vi "Finish.vi"   [LabVIEW 2012]
doc: "This VI is called just before exiting. It is expected to close I/O refnum, save collected data, etc."
uses:
  <vilib>/Rock Robotics/WPI/Compressor/WPI_CompressorGetSetRefNum.vi
  <vilib>/Rock Robotics/WPI/Joystick/WPI_JoystickGetSetRefNum.vi
  <vilib>/Rock Robotics/WPI/RobotDrive/WPI_RobotDriveGetSetRefNum.vi
types:
  T1 = typedef "WPI_ServoDeviceRef.ctl" = cluster{"DeviceStatus":errorcluster, "Digital Module":T2, "PWM Channel":T3, "DeadBand":T4}
  T2 = typedef "FPGA_TypedefDigitalModule.ctl" = enum16{"Digital Module 1", "Digital Module 2"}
  T3 = typedef "FPGA_DIOPWMChannel.ctl" = enum8{"PWM 1", "PWM 2", "PWM 3", "PWM 4", "PWM 5", "PWM 6", "PWM 7", "PWM 8", "PWM 9", "PWM 10", "Invalid"}
  T4 = typedef "WPI_PWMDeadband.ctl" = cluster{"Name":string, "maxPositivePwm":i32, "minPositivePwm":i32, "centerPwm":i32, "maxNegativePwm":i32, "minNegativePwm":i32, "angularRange":u16}
  T5 = typedef "WPI_JoystickDevRef.ctl" = cluster{"Device":T6}
  T6 = typedef "WPI_JoystickDeviceEnum.ctl" = enum16{"USB 1", "USB 2", "USB 3", "USB 4", "Kinect 1", "Kinect 2"}
  T7 = typedef "WPI_RobotDriveDevRef.ctl" = cluster{"DevStatus":errorcluster, "Motors[]":T8[], "Square Inputs":bool, "Max Output":dbl, "Isochronous":bool}
  T8 = typedef "WPI_MotorControlDeviceRef.ctl" = cluster{"DeviceStatus":errorcluster, "Type":enum16{"PWM", "CAN"}, "PWM":cluster{"Digital Module":T2, "PWM Channel":T3, "DeadBand":T4}, "CAN":cluster{"Device Number":u8, "Control Mode":T9, "Semaphore":T10, "Max Vout":dbl}, "Invert":bool, "TransformRef":T11, "InvTransformRef":T11}
  T9 = typedef "WPI_CANJaguar_ControlMode.ctl" = enum8{"Percent VBus", "Current", "Speed", "Position", "Voltage"}
  T10 = typedef "Semaphore RefNum" = refnum<k1>
  T11 = typedef "WPI_PWMTransform_ConPane.ctl" = refnum<vi>
  T12 = typedef "WPI_SolenoidDevRef.ctl" = cluster{"DevStatus":errorcluster, "Solenoid Module":T13, "Forward Solenoid Channel":T14, "Reverse Solenoid Channel":T14}
  T13 = typedef "FPGA_TypedefSolenoidModule.ctl" = enum16{"Solenoid Module 1", "Solenoid Module 2"}
  T14 = typedef "WPI_SolenoidChannel.ctl" = enum8{"Solenoid 1", "Solenoid 2", "Solenoid 3", "Solenoid 4", "Solenoid 5", "Solenoid 6", "Solenoid 7", "Solenoid 8", "Invalid"}
  T15 = typedef "WPI_EncoderDevRef.ctl" = cluster{"DevStatus":errorcluster, "EncoderIndex":T16, "CounterIndex":T17, "DistancePerCount":dbl, "Decoding Type":T18}
  T16 = typedef "FPGA_EncoderIdx.ctl" = enum8{"Enc 0", "Enc 1", "Enc 2", "Enc 3", "Invalid"}
  T17 = typedef "FPGA_CounterCtrSystemIndex.ctl" = enum8{"Ctr 0", "Ctr 1", "Ctr 2", "Ctr 3", "Ctr 4", "Ctr 5", "Ctr 6", "Ctr 7", "Invalid"}
  T18 = typedef "WPI_EncoderType.ctl" = enum16{"1x", "2x", "4x"}
  T19 = typedef "WPI_GyroDevRef.ctl" = cluster{"DevStatus":errorcluster, "Analog Module":T20, "Analog Channel":T21, "Offset":dbl, "Gain (VoltsPerDegree/Second)":dbl}
  T20 = typedef "FPGA_TypedefAnalogModule.ctl" = enum16{"Analog Module 1", "Analog Module 2"}
  T21 = typedef "FPGA_AIChannel.ctl" = enum8{"AI 1", "AI 2", "AI 3", "AI 4", "AI 5", "AI 6", "AI 7", "AI 8", "Invalid"}
  T22 = typedef "WPI_DigitalInputDevRef.ctl" = cluster{"DevStatus":errorcluster, "DIO Channel":T23, "Digital Module":T2}
  T23 = typedef "FPGA_DIOChannel.ctl" = enum8{"DIO 1", "DIO 2", "DIO 3", "DIO 4", "DIO 5", "DIO 6", "DIO 7", "DIO 8", "DIO 9", "DIO 10", "DIO 11", "DIO 12", "DIO 13", "DIO 14", "Invalid"}
  T24 = typedef "WPI_CompressorDevRef.ctl" = cluster{"DevStatus":errorcluster, "DigitalInputDevRef":T22, "RelayDevRef":T25}
  T25 = typedef "WPI_RelayDevRef.ctl" = cluster{"DevStatus":errorcluster, "Relay Channel":T26, "Digital Module":T2, "Relay Direction":T27}
  T26 = typedef "FPGA_DIORelayChannel.ctl" = enum8{"Relay 1", "Relay 2", "Relay 3", "Relay 4", "Relay 5", "Relay 6", "Relay 7", "Relay 8", "Invalid"}
  T27 = typedef "WPI_RelayDirection.ctl" = enum16{"Both directions", "Forward only", "Reverse only"}
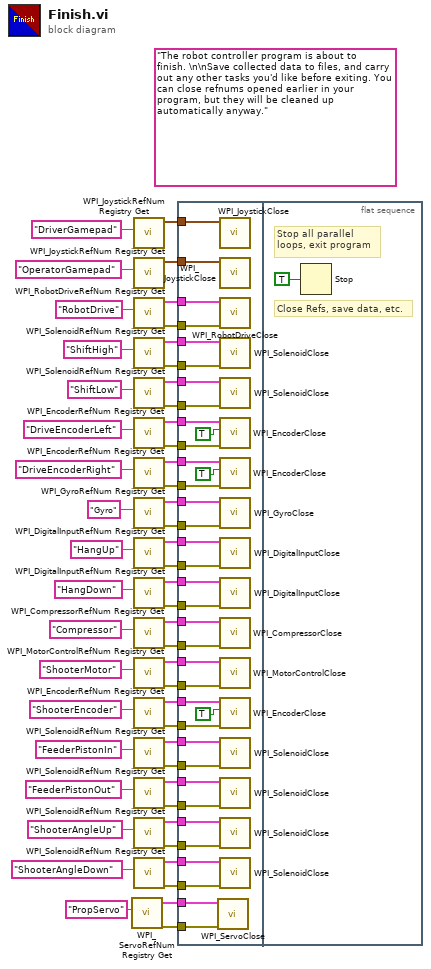
[diagram p0: block diagram]
diagram:
  (unwired) "The robot controller program is about to finish. \n\nSave collected data to files, and carry out any other tasks you'd like before exiting. You can close refnums opened earlier in your program, but they will be cleaned up automatically anyway."
  n1 = call <vilib>:"WPI_ServoRefNum Registry Get.vi"("refnum name"="PropServo") -> ("error out"=w1:errorcluster, "ServoDeviceRef"=w2:T1)  [unwired: 9 in]
  n2 = call <vilib>:"WPI_JoystickRefNum Registry Get.vi"("refnum name"="DriverGamepad") -> ("JoystickDevRef"=w35:T5)  [unwired: 1 in, 9 out]
  n3 = call <vilib>:"WPI_JoystickRefNum Registry Get.vi"("refnum name"="OperatorGamepad") -> ("JoystickDevRef"=w34:T5)  [unwired: 1 in, 9 out]
  n4 = call <vilib>:"WPI_RobotDriveRefNum Registry Get.vi"("refnum name"="RobotDrive") -> ("error out"=w31:errorcluster, "RobotDriveDevRef"=w33:T7)  [unwired: 1 in, 8 out]
  n5 = call <vilib>:"WPI_SolenoidRefNum Registry Get.vi"("refnum name"="ShiftHigh") -> ("error out"=w30:errorcluster, "SolenoidDevRef"=w32:T12)  [unwired: 9 in]
  n6 = call <vilib>:"WPI_SolenoidRefNum Registry Get.vi"("refnum name"="ShiftLow") -> ("error out"=w28:errorcluster, "SolenoidDevRef"=w29:T12)  [unwired: 9 in]
  n7 = call <vilib>:"WPI_EncoderRefNum Registry Get.vi"("refnum name"="DriveEncoderLeft") -> ("error out"=w26:errorcluster, "EncoderDevRef"=w27:T15)  [unwired: 9 in]
  n8 = call <vilib>:"WPI_EncoderRefNum Registry Get.vi"("refnum name"="DriveEncoderRight") -> ("error out"=w22:errorcluster, "EncoderDevRef"=w23:T15)  [unwired: 9 in]
  n9 = call <vilib>:"WPI_GyroRefNum Registry Get.vi"("refnum name"="Gyro") -> ("error out"=w24:errorcluster, "GyroDevRef"=w25:T19)  [unwired: 9 in]
  n10 = call <vilib>:"WPI_DigitalInputRefNum Registry Get.vi"("refnum name"="HangUp") -> ("error out"=w20:errorcluster, "DigitalInputDevRef"=w21:T22)  [unwired: 9 in]
  n11 = call <vilib>:"WPI_DigitalInputRefNum Registry Get.vi"("refnum name"="HangDown") -> ("error out"=w18:errorcluster, "DigitalInputDevRef"=w19:T22)  [unwired: 9 in]
  n12 = call <vilib>:"WPI_CompressorRefNum Registry Get.vi"("refnum name"="Compressor") -> ("error out"=w16:errorcluster, "CompressorDevRef"=w17:T24)  [unwired: 9 in]
  n13 = call <vilib>:"WPI_MotorControlRefNum Registry Get.vi"("refnum name"="ShooterMotor") -> ("error out"=w14:errorcluster, "MotorControlDevRef"=w15:T8)  [unwired: 9 in]
  n14 = call <vilib>:"WPI_EncoderRefNum Registry Get.vi"("refnum name"="ShooterEncoder") -> ("error out"=w12:errorcluster, "EncoderDevRef"=w13:T15)  [unwired: 9 in]
  n15 = call <vilib>:"WPI_SolenoidRefNum Registry Get.vi"("refnum name"="FeederPistonIn") -> ("error out"=w10:errorcluster, "SolenoidDevRef"=w11:T12)  [unwired: 9 in]
  n16 = call <vilib>:"WPI_SolenoidRefNum Registry Get.vi"("refnum name"="FeederPistonOut") -> ("error out"=w8:errorcluster, "SolenoidDevRef"=w9:T12)  [unwired: 9 in]
  n17 = call <vilib>:"WPI_SolenoidRefNum Registry Get.vi"("refnum name"="ShooterAngleUp") -> ("error out"=w6:errorcluster, "SolenoidDevRef"=w7:T12)  [unwired: 9 in]
  n18 = call <vilib>:"WPI_SolenoidRefNum Registry Get.vi"("refnum name"="ShooterAngleDown") -> ("error out"=w4:errorcluster, "SolenoidDevRef"=w5:T12)  [unwired: 9 in]
  n19 = flat-sequence {
    tunnel: w35 -> [w89]
    tunnel: w34 -> [w88]
    tunnel: w33 -> [w87]
    tunnel: w32 -> [w86]
    tunnel: w31 -> [w85]
    tunnel: w30 -> [w84]
    tunnel: w29 -> [w83]
    tunnel: w28 -> [w82]
    tunnel: w27 -> [w81]
    tunnel: w26 -> [w80]
    tunnel: w25 -> [w76]
    tunnel: w24 -> [w75]
    tunnel: w23 -> [w74]
    tunnel: w22 -> [w73]
    tunnel: w21 -> [w72]
    tunnel: w20 -> [w71]
    tunnel: w19 -> [w70]
    tunnel: w18 -> [w69]
    tunnel: w17 -> [w68]
    tunnel: w16 -> [w67]
    tunnel: w15 -> [w66]
    tunnel: w14 -> [w65]
    tunnel: w13 -> [w64]
    tunnel: w12 -> [w63]
    tunnel: w11 -> [w62]
    tunnel: w10 -> [w61]
    tunnel: w9 -> [w60]
    tunnel: w8 -> [w59]
    tunnel: w7 -> [w58]
    tunnel: w6 -> [w57]
    tunnel: w5 -> [w56]
    tunnel: w4 -> [w55]
    tunnel: w2 -> [w54]
    tunnel: w1 -> [w53]
    frame #0 {
      n20 = call <vilib>:"WPI_ServoClose.vi"("error in (no error)"=w53, "MotorControlDevRef"=w54) -> ()  [unwired: 9 in, 1 out]
      n21 = call <vilib>:"WPI_JoystickClose.vi"("JoystickDevRef"=w89) -> ()  [unwired: 11 out]
      n22 = call <vilib>:"WPI_JoystickClose.vi"("JoystickDevRef"=w88) -> ()  [unwired: 11 out]
      n23 = call <vilib>:"WPI_RobotDriveClose.vi"("error in (no error)"=w85, "RobotDriveDevRef"=w87) -> ()  [unwired: 10 out]
      n24 = call <vilib>:"WPI_SolenoidClose.vi"("error in (no error)"=w84, "SolenoidDevRef"=w86) -> ()  [unwired: 9 in, 1 out]
      n25 = call <vilib>:"WPI_SolenoidClose.vi"("error in (no error)"=w82, "SolenoidDevRef"=w83) -> ()  [unwired: 9 in, 1 out]
      n26 = call <vilib>:"WPI_EncoderClose.vi"("error in (no error)"=w80, "Close Dependencies"=TRUE, "EncoderDevRef"=w81) -> ()  [unwired: 8 in, 1 out]
      n27 = call <vilib>:"WPI_EncoderClose.vi"("error in (no error)"=w73, "Close Dependencies"=TRUE, "EncoderDevRef"=w74) -> ()  [unwired: 8 in, 1 out]
      n28 = call <vilib>:"WPI_GyroClose.vi"("error in (no error)"=w75, "GyroDevRef"=w76) -> ()  [unwired: 9 in, 1 out]
      n29 = call <vilib>:"WPI_DigitalInputClose.vi"("error in (no error)"=w71, "DigitalInputDevRef"=w72) -> ()  [unwired: 9 in, 1 out]
      n30 = call <vilib>:"WPI_DigitalInputClose.vi"("error in (no error)"=w69, "DigitalInputDevRef"=w70) -> ()  [unwired: 9 in, 1 out]
      n31 = call <vilib>:"WPI_CompressorClose.vi"("error in (no error)"=w67, "CompressorDevRef"=w68) -> ()  [unwired: 9 in, 1 out]
      n32 = call <vilib>:"WPI_MotorControlClose.vi"("error in (no error)"=w65, "MotorControlDevRef"=w66) -> ()  [unwired: 9 in, 1 out]
      n33 = call <vilib>:"WPI_EncoderClose.vi"("error in (no error)"=w63, "Close Dependencies"=TRUE, "EncoderDevRef"=w64) -> ()  [unwired: 8 in, 1 out]
      n34 = call <vilib>:"WPI_SolenoidClose.vi"("error in (no error)"=w61, "SolenoidDevRef"=w62) -> ()  [unwired: 9 in, 1 out]
      n35 = call <vilib>:"WPI_SolenoidClose.vi"("error in (no error)"=w59, "SolenoidDevRef"=w60) -> ()  [unwired: 9 in, 1 out]
      n36 = call <vilib>:"WPI_SolenoidClose.vi"("error in (no error)"=w57, "SolenoidDevRef"=w58) -> ()  [unwired: 9 in, 1 out]
      n37 = call <vilib>:"WPI_SolenoidClose.vi"("error in (no error)"=w55, "SolenoidDevRef"=w56) -> ()  [unwired: 9 in, 1 out]
    }
    frame #1 {
      # "Close Refs, save data, etc."
      # "Stop all parallel\nloops, exit program"
      n38 = Stop(stop? (T)=TRUE ("Quit")) -> ()
    }
  }
